vi "Update Addon To Latest Version.vi"(8 "error in (no error)":errorcluster, 11 "Device Item Ref in":T1 format="%.0x") -> (0 "error out":errorcluster, 3 "Device Item Ref out":T1 format="%.0x")   [LabVIEW 2019, in "Instrument Addon Shared.lvlib"]
uses:
  Instrument Addon Shared.lvlib
  <vilib>/NI VeriStand/Custom Device API/Custom Device Item Ref.ctl
  <vilib>/NI VeriStand/Custom Device API/Custom Device Channel.ctl
  <vilib>/NI VeriStand/Custom Device API/Custom Device Channel Type.ctl
  NationalInstruments.VeriStand.SystemDefinitionAPI
  Constants.vi
  <vilib>/NI/NI VeriStand Advanced SysDef API/_SubVIs/SysDef.Search.GUIDs.vi
  <vilib>/NI VeriStand/Custom Device API/Custom Device API.lvlib
  <vilib>/NI/NI VeriStand Advanced SysDef API/SysDef API/Advanced System Definition.lvlib
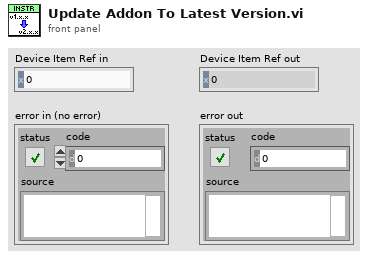
[diagram p1: front panel]
types:
  T1 = typedef "Custom Device API.lvlib/Custom Device Item Ref.ctl" = u64
  T2 = typedef "Custom Device API.lvlib/Custom Device Channel.ctl" = cluster{"Type":T3, "Units":string, "Default Value":dbl, "Faultable":bool, "Scalable":bool}
  T3 = typedef "Custom Device API.lvlib/Custom Device Channel Type.ctl" = enum16{"Input", "Output"}
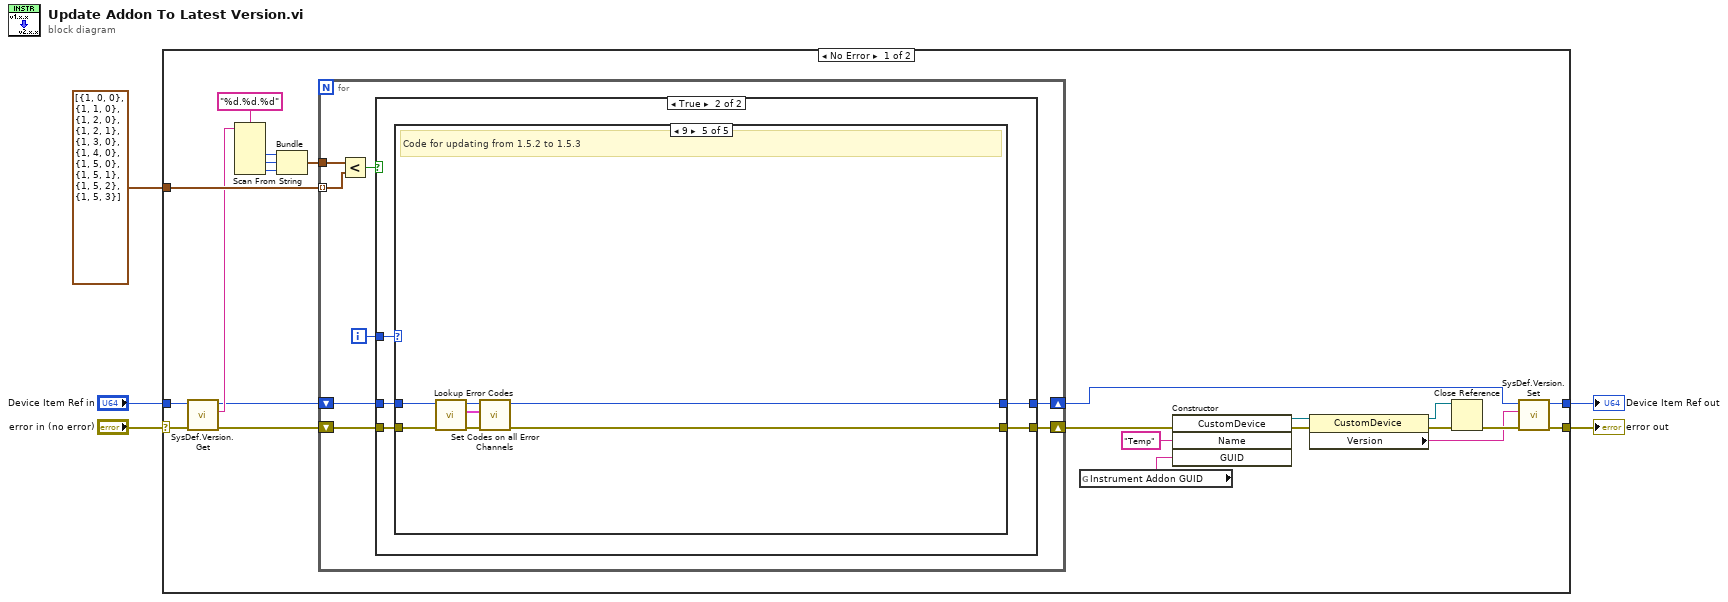
[diagram p0: block diagram]
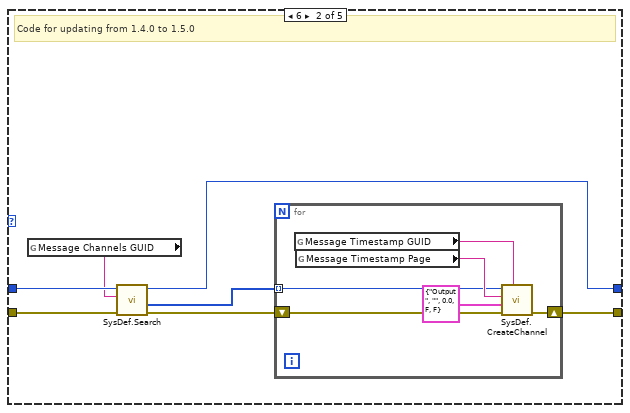
[diagram p4: hidden frame]
diagram:
  n1 = case shown="No Error" "error in (no error)" {
    selector: "error in (no error)" -> [w11 w71]
    tunnel: [w20 w71] -> w4
    tunnel: "Device Item Ref in" -> [w10 w70]
    tunnel: [w21 w70] -> w5
    tunnel: cluster{i32, i32, i32}[] [{1, 0, 0}, {1, 1, 0}, {1, 2, 0}, {1, 2, 1}, {1, 3, 0}, {1, 4, 0}, {1, 5, 0}, {1, 5, 1}, {1, 5, 2}, {1, 5, 3}] -> [w28 _]
    frame No Error {
      n2 = call <vilib>:"SysDef.Version.Get.vi"("error in (no error)"=w11, "nodeID"=w10) -> ("error out"=w7:errorcluster, "Version"=w14:string, "nodeID out"=w6:u64)  [unwired: 7 in]
      n3 = Scan From String(format string="%d.%d.%d", input string=w14) -> (output 1=w13:i32, output 2=w12:i32, output 3=w15:i32)  [unwired: 5 in, 3 out]
      n4 = Bundle(w13, w12, w15) -> (w8:cluster{i32, i32, i32})  [unwired: 1 in]
      n5 = for {
        shift-right: [w35] -> w19
        shift-left: w7 -> [w30]
        shift-right: [w34] -> w18
        shift-left: w6 -> [w29]
        tunnel: w28 -> [w31] mode=indexing
        tunnel: w8 -> [w32]
        i -> [w33]
        n6 = Less?(x=w32, y=w31) -> (x < y?=w36:bool)
        n7 = case shown="True" w36 {
          tunnel: w30 -> [w38 w43]
          tunnel: [w38 w42] -> w35
          tunnel: w29 -> [w37 w39]
          tunnel: [w37 w40] -> w34
          tunnel: w33 -> [_ w41]
          frame False {
          }
          frame True {
            n8 = case shown="9" w41 {
              tunnel: w43 -> [w45 w51 w60 w62 w65]
              tunnel: [w45 w46 w60 w62 w69] -> w42
              tunnel: [w44 w47 w59 w61 w68] -> w40
              tunnel: w39 -> [w44 w52 w59 w61 w67]
              frame Default {
              }
              frame 6 {
                # "Code for updating from 1.4.0 to 1.5.0"
                n9 = global read "Constants.vi" "Message Channels GUID"() -> (w50:string)
                n10 = call-poly <vilib>:"SysDef.Search.vi"("error in (no error)"=w51, "GUID"=w50, "nodeID"=w52) -> ("error out"=w49:errorcluster, "Values Out"=w48:u64[], "nodeID out"=w47:u64)  [unwired: 5 in, 1 out]
                n11 = for {
                  tunnel: w48 -> [w53] mode=indexing
                  shift-right: [w54] -> w46
                  shift-left: w49 -> [w55]
                  n12 = global read "Constants.vi" "Message Timestamp GUID"() -> (w57:string)
                  n13 = global read "Constants.vi" "Message Timestamp Page"() -> (w58:string)
                  n14 = call <vilib>:"SysDef.CreateChannel.vi"("GUID"=w57, "error in (no error)"=w55, "Channel"=T2 {"Type"=enum."Output", "Units"="", "Default Value"=0.0, "Faultable"=FALSE, "Scalable"=FALSE}, "Name"=w58, "nodeID"=w53) -> ("error out"=w54:errorcluster)  [unwired: 3 in, 3 out]
                }
              }
              frame 7 {
                # "Code for updating from 1.5.0 to 1.5.1"
              }
              frame 8 {
                # "Code for updating from 1.5.1 to 1.5.2"
              }
              frame 9 {
                # "Code for updating from 1.5.2 to 1.5.3"
                n15 = call "Lookup Error Codes.vi"("error in (no error)"=w65, "Node Ptr"=w67) -> ("error out"=w64:errorcluster, "Error Codes"=w63:cluster{"Code":i32, "String":string}[], "Node Ptr out"=w66:u64)  [unwired: 7 in]
                n16 = call "Set Codes on all Error Channels.vi"("error in (no error)"=w64, "Error Codes"=w63, "Node Ptr in"=w66) -> ("error out"=w69:errorcluster, "Section Ref out"=w68:T1)  [unwired: 7 in]
              }
            }
          }
        }
      }
      n17 = global read "Constants.vi" "Instrument Addon GUID"() -> (w16:string)
      n18 = constructor class="CustomDevice"(error in=w19, "Name"="Temp", "GUID"=w16) -> (reference out=w27:refnum<k24>, error out=w26:errorcluster)  [unwired: 2 in, 3 out]
      n19 = property class="CustomDevice"(reference=w27, error in=w26) -> (reference out=w24:refnum<k24>, error out=w25:errorcluster, "Version"=w22:string)
      n20 = Close Reference(reference=w24, error in (no error)=w25) -> (error out=w23:errorcluster)
      n21 = call <vilib>:"SysDef.Version.Set.vi"("error in (no error)"=w23, "Version"=w22, "nodeID"=w18) -> ("error out"=w20:errorcluster, "nodeID out"=w21:u64)  [unwired: 7 in]
    }
    frame Error {
    }
  }
  "Device Item Ref out" <- w5
  "error out" <- w4
